vi "Run.vi"(8 "error in (no error)":errorcluster, 11 "Data Sharing Plugin in":refnum<class "Plugin.lvclass">) -> (0 "error out":errorcluster, 3 "Data Sharing Plugin out":refnum<class "Plugin.lvclass">)   [LabVIEW 2016, in "Plugin.lvclass"]
uses:
  Plugin.lvclass
  Plugin.lvclass/Plugin.ctl
  Plugin Runtime/Plugin Runtime.lvclass
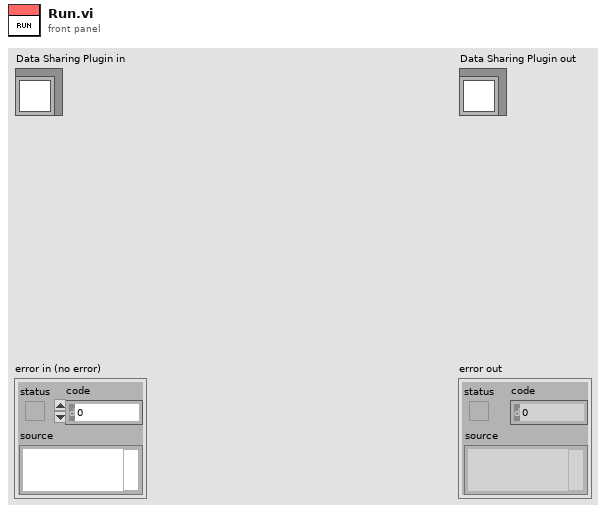
[diagram p1: front panel]
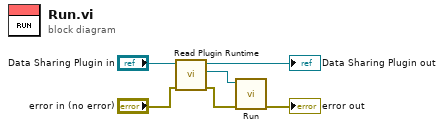
[diagram p0: block diagram]
diagram:
  n1 = call "Read Plugin Runtime.vi"("error in (no error)"="error in (no error)", "Data Sharing Plugin in"="Data Sharing Plugin in") -> ("error out"=w5:errorcluster, "Data Sharing Plugin Runtime"=w6:refnum<class "Plugin Runtime.lvclass">, "Data Sharing Plugin out"=→"Data Sharing Plugin out":refnum<class "Plugin.lvclass">)  [unwired: 7 in]
  n2 = call-dynamic "Run.vi"("error in (no error)"=w5, "Data Sharing Plugin Runtime in"=w6) -> ("error out"=→"error out":errorcluster)  [unwired: 8 in, 1 out]
